vi "Decompress.vi"(8 "error in (no error)":errorcluster, 10 "compressed data":string, 11 "lvzstd in":refnum<class "lvzstd.lvclass">) -> (0 "error out":errorcluster, 2 "uncompressed data":string, 3 "lvzstd out":refnum<class "lvzstd.lvclass">)   [LabVIEW 2020, in "lvzstd.lvlib" / "lvzstd.lvclass"]
uses:
  lvzstd.lvclass
  lvzstd.lvclass/lvzstd.ctl
  <vilib>/Utility/error.llb/Error Cluster From Error Code.vi
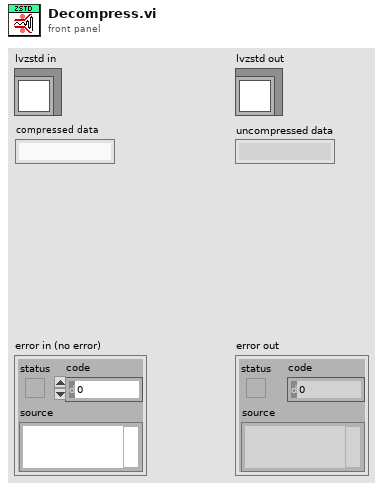
[diagram p1: front panel]
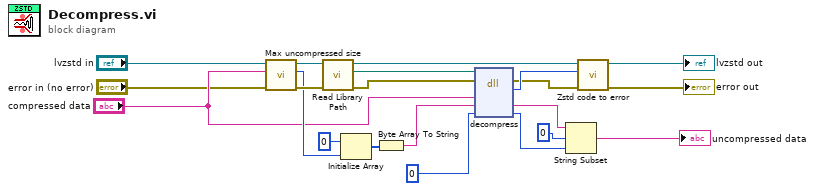
[diagram p0: block diagram]
diagram:
  n1 = call-dynamic "Max uncompressed size.vi"("error in (no error)"="error in (no error)", "srcHandle"="compressed data", "lvzstd in"="lvzstd in") -> ("error out"=w9:errorcluster, "uncompressed size"=w8:i32, "lvzstd out"=w10:refnum<class "lvzstd.lvclass">)  [unwired: 6 in]
  n2 = call "Read Library Path.vi"("error in (no error)"=w9, "lvzstd in"=w10) -> ("error out"=w20:errorcluster, "Library Path"=w21:path, "lvzstd out"=w13:refnum<class "lvzstd.lvclass">)  [unwired: 7 in]
  n3 = Initialize Array(u8 0, w8) -> (w18:u8[])
  n4 = Byte Array To String(unsigned byte array=w18) -> (string=w17:string)
  n5 = dll-call lib="?" fn="decompress"(path in=w21, error in=w20, "srcHandle"="compressed data", "dstHandle"=w17, "uncompressedSize"=0 ("compressedSize")) -> (error out=w14:errorcluster, "return type"=w15:i32, "dstHandle"=w11:string, "uncompressedSize"=w4:i32)  [unwired: 2 in, 1 out]
  n6 = String Subset(string=w11, offset (0)=0, length (rest)=w4) -> (substring=→"uncompressed data":string)
  n7 = call "Zstd code to error.vi"("error in"=w14, "Error code"=w15, "lvzstd in"=w13) -> ("error in (no error)"=→"error out":errorcluster, "lvzstd out"=→"lvzstd out":refnum<class "lvzstd.lvclass">)  [unwired: 7 in]
